vi "nirviSimLinearInterp.vi"(0 "y0":dbl, 2 "y1":dbl, 3 "x (fractional)":dbl) -> (7 "y":dbl)   [LabVIEW 2020]
panel:
  # "x can be any length with 16-bit fractional portion"
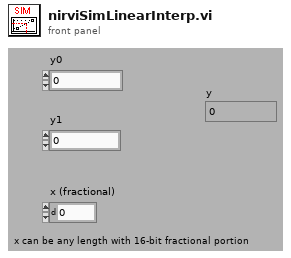
[diagram p1: front panel]
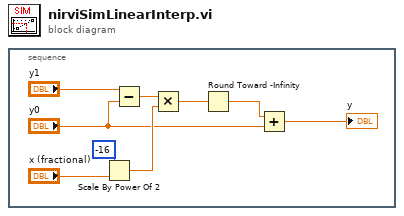
[diagram p0: block diagram]
diagram:
  n1 = stacked-sequence {
    frame #0 {
      n2 = Scale By Power Of 2(n=-16, x="x (fractional)") -> (x*2^n=w7:dbl)
      n3 = Subtract(x="y1", y="y0") -> (x-y=w9:dbl)
      n4 = Multiply(x=w9, y=w7) -> (x*y=w6:dbl)
      n5 = Round Toward -Infinity(1:w6) -> (0:w5:dbl)
      n6 = Add(x=w5, y="y0") -> (x+y=→"y":dbl)
    }
  }
